vi "运维调试_采配水.vi"() -> ()   [LabVIEW 2016, in "PLC.lvlib"]
uses:
  PLC.lvlib
  <vilib>/Plasmionique/MB Master/MB_Master/MB_Master.lvclass
  <vilib>/Utility/miscctls.llb/LVPointTypeDef.ctl
  <vilib>/Plasmionique/MB Master/MB_Master_Serial/MB_Master_Serial.lvclass
  C:/Program Files (x86)/National Instruments/LabVIEW 2016/vi.lib/Plasmionique/MB Master/MB_Master/MB_Master.lvclass
  <vilib>/Plasmionique/MB Master/MB Master.lvlib
panel:
  out "R113":i16 caption="储水时间设定"
  out "R25":i16
  in  "V14NC":bool
  out "R24":i16
  in  "V14NO":bool
  out "X2":bool caption="X1"
  out "采配水版本号":string
  out "R23":i16 caption="清洗频次计数"
  out "R112":i16 caption="清洗频次设定"
  out "R22":i16
  in  "V13NC":bool
  out "R111":i16 caption="排液时间"
  out "通讯故障":bool
  out "R21":i16
  in  "V13NO":bool
  out "R20":i16
  in  "M1-2":bool
  in  "潜水泵工作模式":u16(ring) items=["泵1单泵单管路", "泵2单泵单管路", "双泵双管路"]
  out "X11":bool caption="废液报警"
  out "X10":bool caption="自来水检测"
  out "X9":bool caption="泵2过载报警"
  out "X8":bool caption="泵1过载报警"
  out "X7":bool caption="断电检测"
  out "X6":bool caption="开门检测"
  out "X5":bool caption="烟雾检测"
  out "X4":bool caption="漏水检测"
  out "X3":bool caption="进样检测"
  out "X1":bool
  out "X0":bool caption="采样池液位开关"
  out "R109":i16 caption="配水时间"
  out "集成报警信息":string
  out "R108":i16 caption="自来水报警"
  out "R107":i16 caption="采水池液位报警设置"
  out "R106":i16 caption="进样超时设置"
  out "R105":i16 caption="二级清洗时间"
  out "R104":i16 caption="一级清洗时间"
  out "R103":i16 caption="外部管路清洗时间"
  out "R102":i16 caption="静置沉淀时间"
  out "R101":i16 caption="内部管路润洗时间"
  out "R100":i16 caption="外部管路润洗时间"
  out "R2":i16
  out "R1":i16
  out "多列列表框":i32(listbox)
  out "R19":i16
  in  "V6":bool
  out "R18":i16
  in  "V5":bool
  out "R17":i16
  in  "V4":bool
  out "R16":i16
  in  "V3":bool
  out "R15":i16
  in  "V2":bool
  out "R14":i16
  in  "M2":bool
  out "R13":i16
  in  "V1":bool
  out "R12":i16
  in  "M1-1":bool
  in  "返回":bool
  in  "参数设置":bool
  in  "单步启动":bool
  in  "启动":bool
  in  "停止":bool
  # "S"
  # "次"
  # "次"
  # "S"
  # "S"
  # "S"
  # "S"
  # "S"
  # "S"
  # "S"
  # "S"
  # "S"
  # "S"
  # "S"
  # "单步计时："
  # "s"
  # "流程计时："
  # "s"
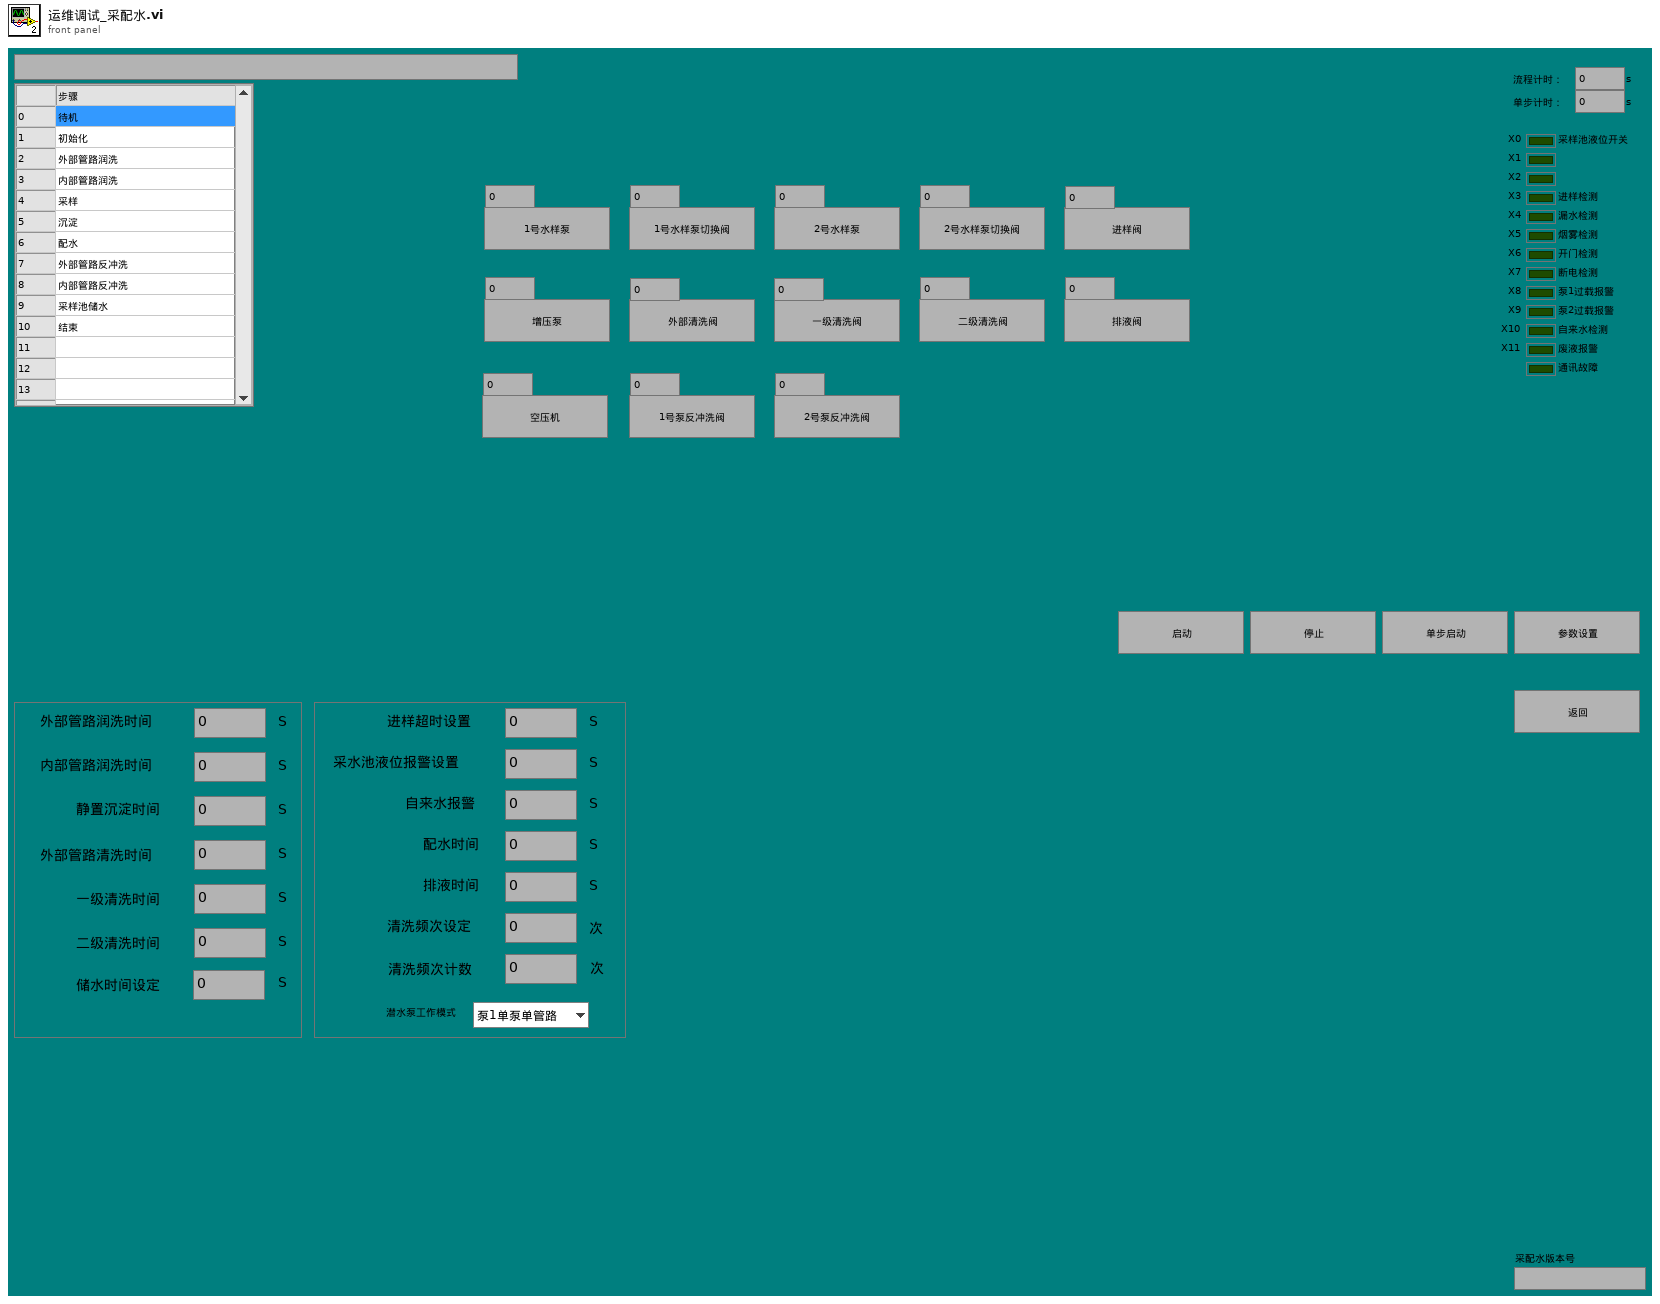
[diagram p1: front panel]
types:
  T1 = typedef "LVPointTypeDef.ctl" = cluster{"Horizontal":i16, "Vertical":i16}
  T2 = cluster{"时间标识":timestamp, "设备":string, "日志信息":string}
  T3 = cluster{"R0":i16, "R1":i16, "R2":i16, "R3":i16, "R4":i16, "R5":i16, "R6":i16, "R7":i16, "R8":i16, "R9":i16, "R10":i16, "R11":i16, "R12":i16, "R13":i16, "R14":i16, "R15":i16, "R16":i16, "R17":i16, "R18":i16, "R19":i16, "R20":i16, "R21":i16, "R22":i16, "R23":i16, "R24":i16, "R25":i16}
  T4 = cluster{"seconds since 1Jan1904":timestamp, "table输入":string, string, "table输入":string}
  T5 = cluster{"时间标识":timestamp, "设备":string, "日志信息":string, "流程参数":string}
  T6 = cluster{"命令":string, cluster{"starting address":u16, "holding register value":u16}}
  T7 = cluster{"CODCr":cluster{"启动测量模式":cluster{"测量模式":enum16{"水样测量", "标样核查", "零点核查", "加标回收", "平行样", "校零", "校标"}}, "确定按钮":bool}, "参数启用":cluster{"多参数":bool, "CODMn":bool, "总磷总氮":bool, "氨氮":bool, "CODcr":bool}}
  T8 = enum16{"水样测量", "标样核查", "零点核查", "加标回收", "平行样", "校零", "校标"}
  T9 = cluster{"命令":string, "数据":cluster{"starting address":u16, "holding register value":u16}}
  T10 = cluster{"命令":string, "数据":cluster{"starting address":u16, "holding register values":u16[]}}
  T11 = cluster{"命令":string, "data":cluster{"starting address":u16, "coil values":bool[]}}
  T12 = cluster{"多参数":bool, "CODMn":bool, "总磷总氮":bool, "氨氮":bool, "CODcr":bool}
  T13 = enum32{"Bad", "Idle", "Run top level", "Running"}
  T14 = cluster{"baud rate (bps)":u32, "stop bits":u16, "parity":u16, "flow control":u16, "timeout":u32, "retries":i32}
  T15 = cluster{"starting address":u16, "holding register values":u16[]}
  T16 = cluster{"starting address":u16, "holding register value":u16}
  T17 = cluster{"starting address":u16, "coil values":bool[]}
  T18 = cluster{"Registers[0]":u16, "Registers[1]":u16, "Registers[2]":u16, "Registers[3]":u16, "Registers[4]":u16, "Registers[5]":u16, "Registers[6]":u16, "Registers[7]":u16, "Registers[8]":u16, "Registers[9]":u16, "Registers[10]":u16, "Registers[11]":u16, "Registers[12]":u16, "Registers[13]":u16, "Registers[14]":u16, "Registers[15]":u16, "Registers[16]":u16, "Registers[17]":u16, "Registers[18]":u16, "Registers[19]":u16, "Registers[20]":u16, "Registers[21]":u16, "Registers[22]":u16, "Registers[23]":u16, "Registers[24]":u16, "Registers[25]":u16}
  T19 = cluster{"Registers[0]":u16, "Registers[1]":u16, "Registers[2]":u16, "Registers[3]":u16, "Registers[4]":u16, "Registers[5]":u16}
  T20 = cluster{"Registers[0]":u16, "Registers[1]":u16, "Registers[2]":u16, "Registers[3]":u16, "Registers[4]":u16, "Registers[5]":u16, "Registers[6]":u16, "Registers[7]":u16, "Registers[8]":u16, "Registers[9]":u16, "Registers[10]":u16, "Registers[11]":u16, "Registers[12]":u16, "Registers[13]":u16, "Registers[14]":u16, "Registers[15]":u16, "Registers[16]":u16, "Registers[17]":u16, "Registers[18]":u16, "Registers[19]":u16}
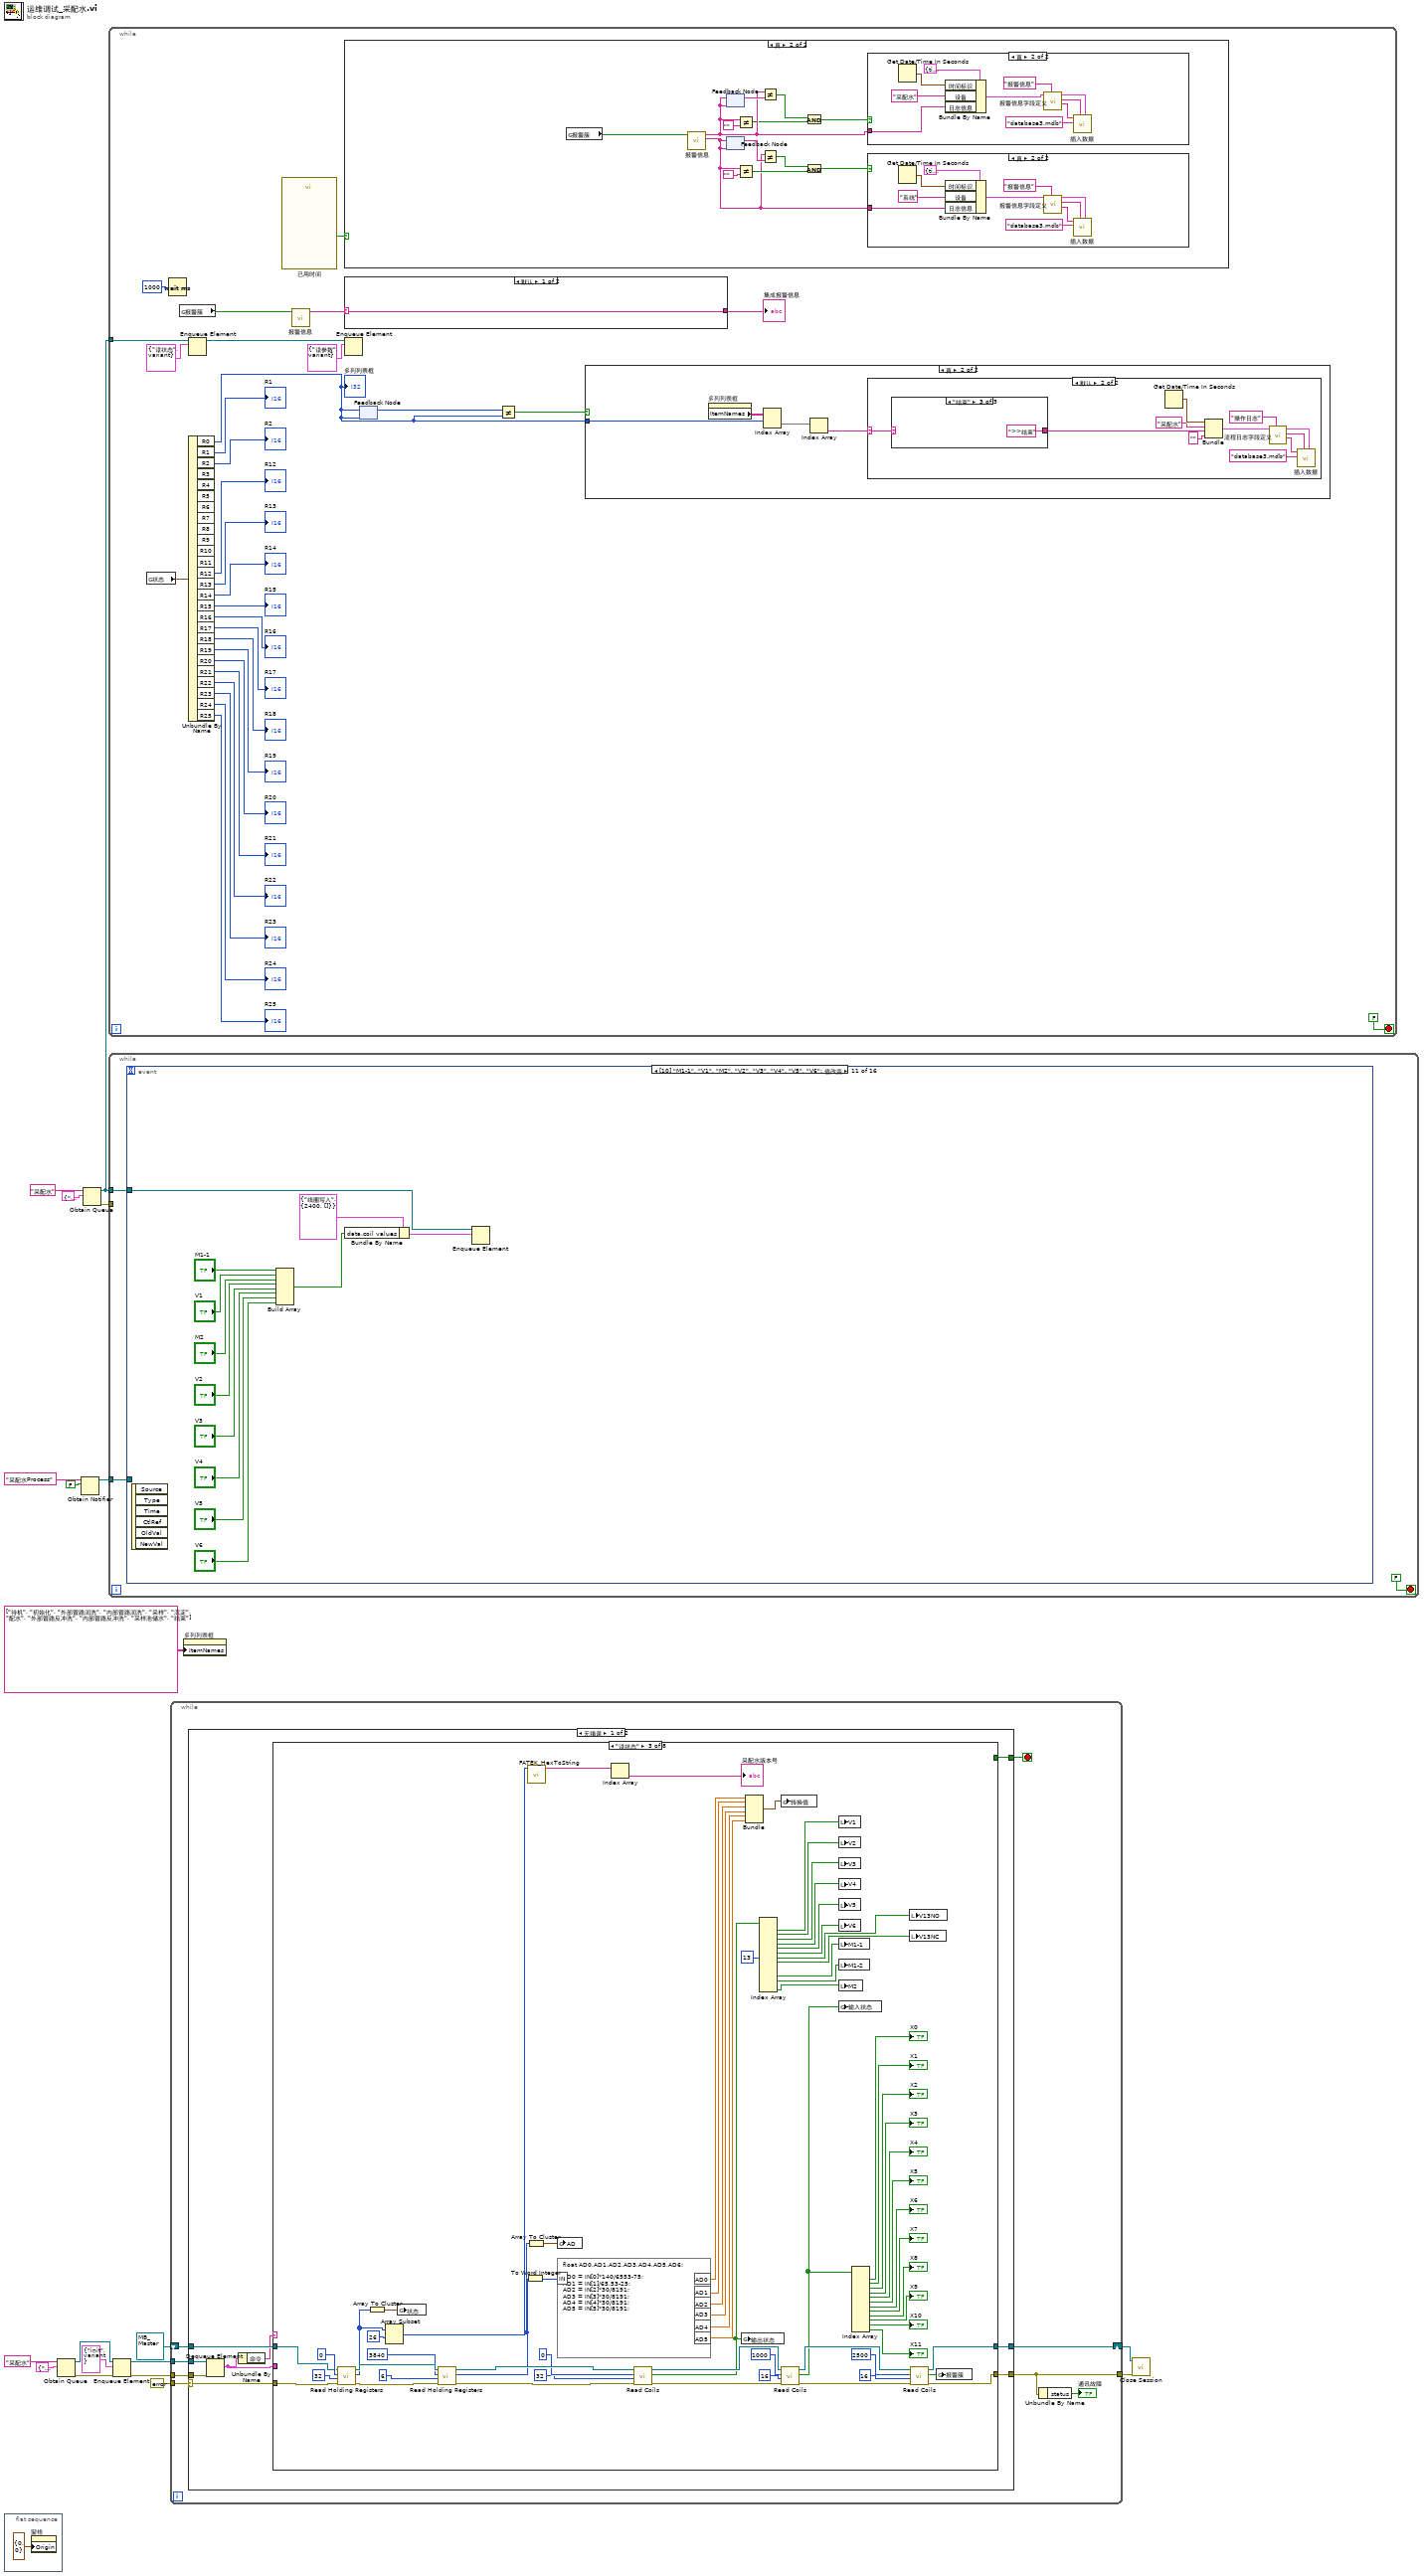
[diagram p0: block diagram]
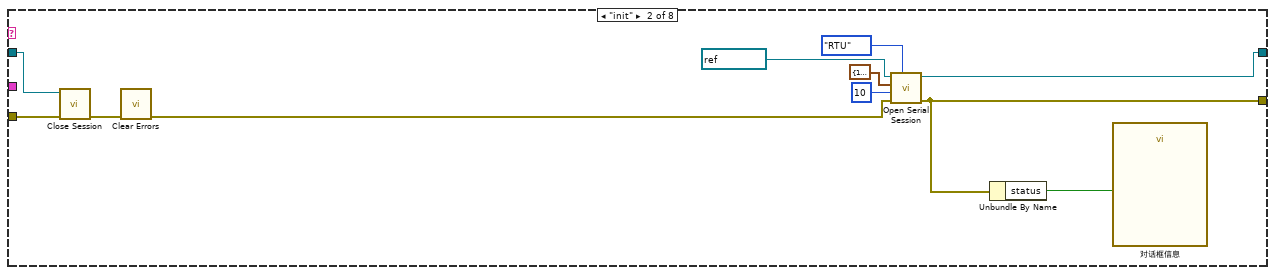
[diagram p3: hidden frame]
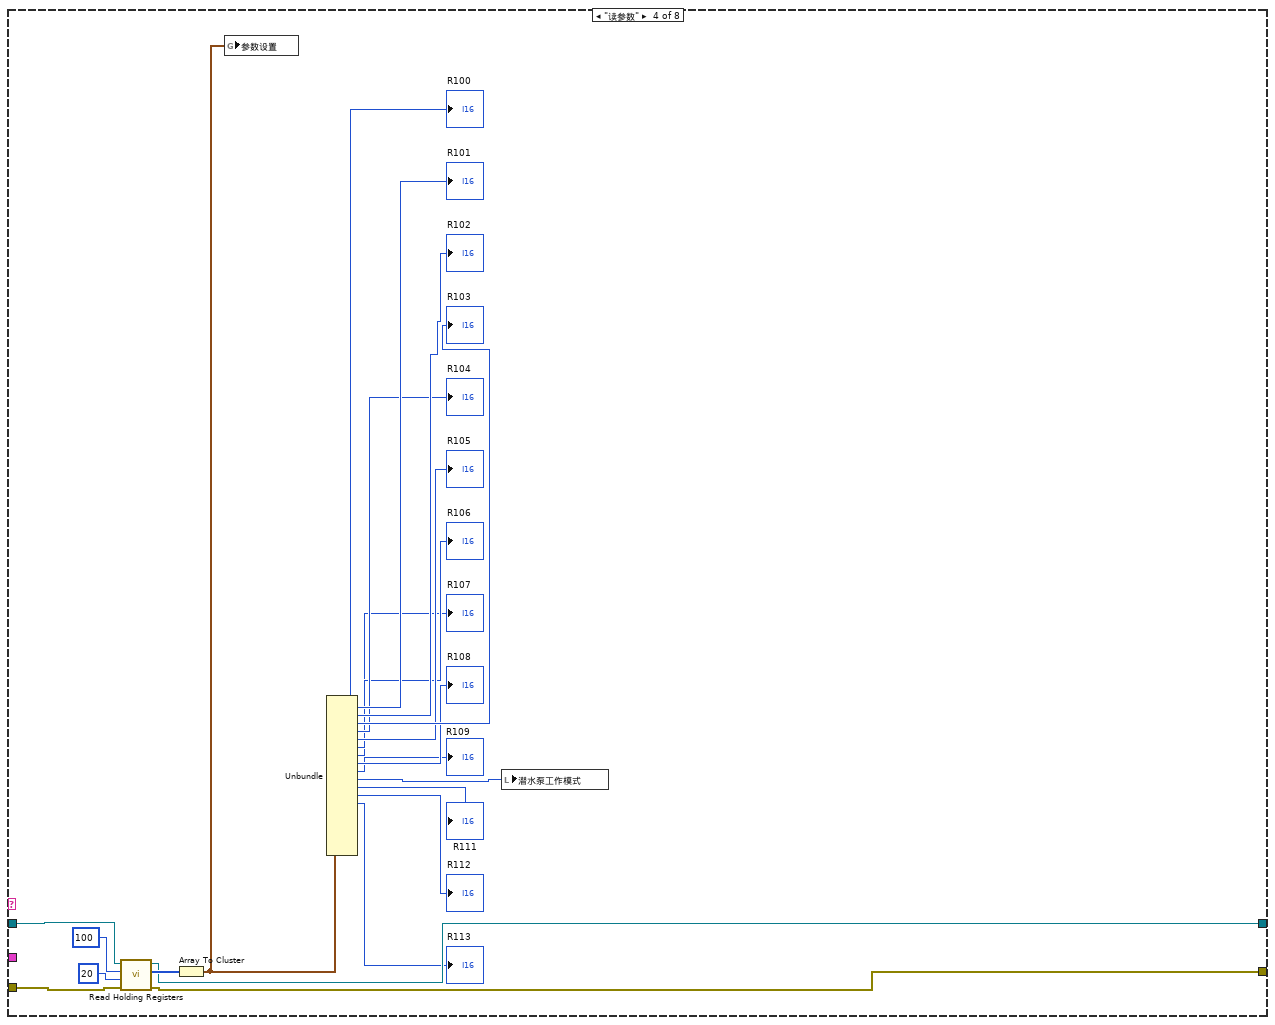
[diagram p4: hidden frame]
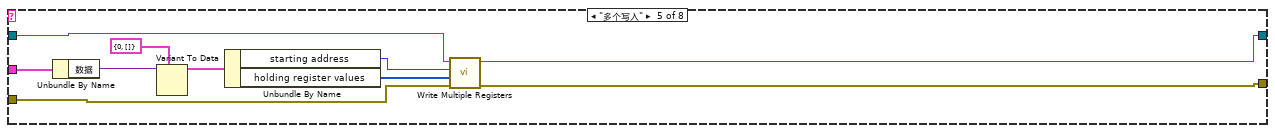
[diagram p5: hidden frame]
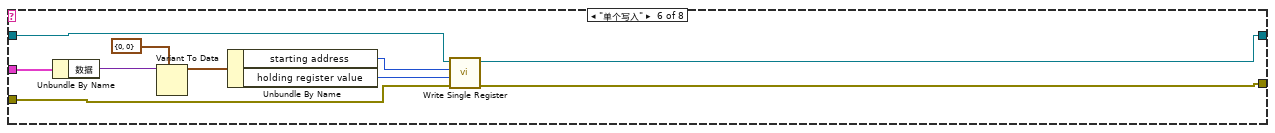
[diagram p6: hidden frame]
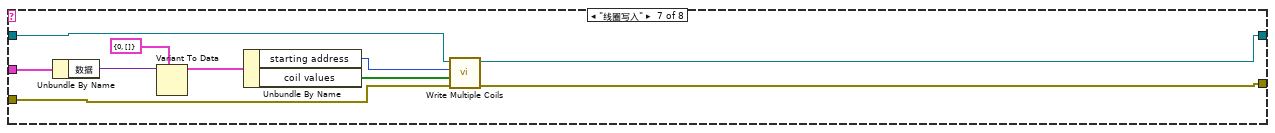
[diagram p7: hidden frame]
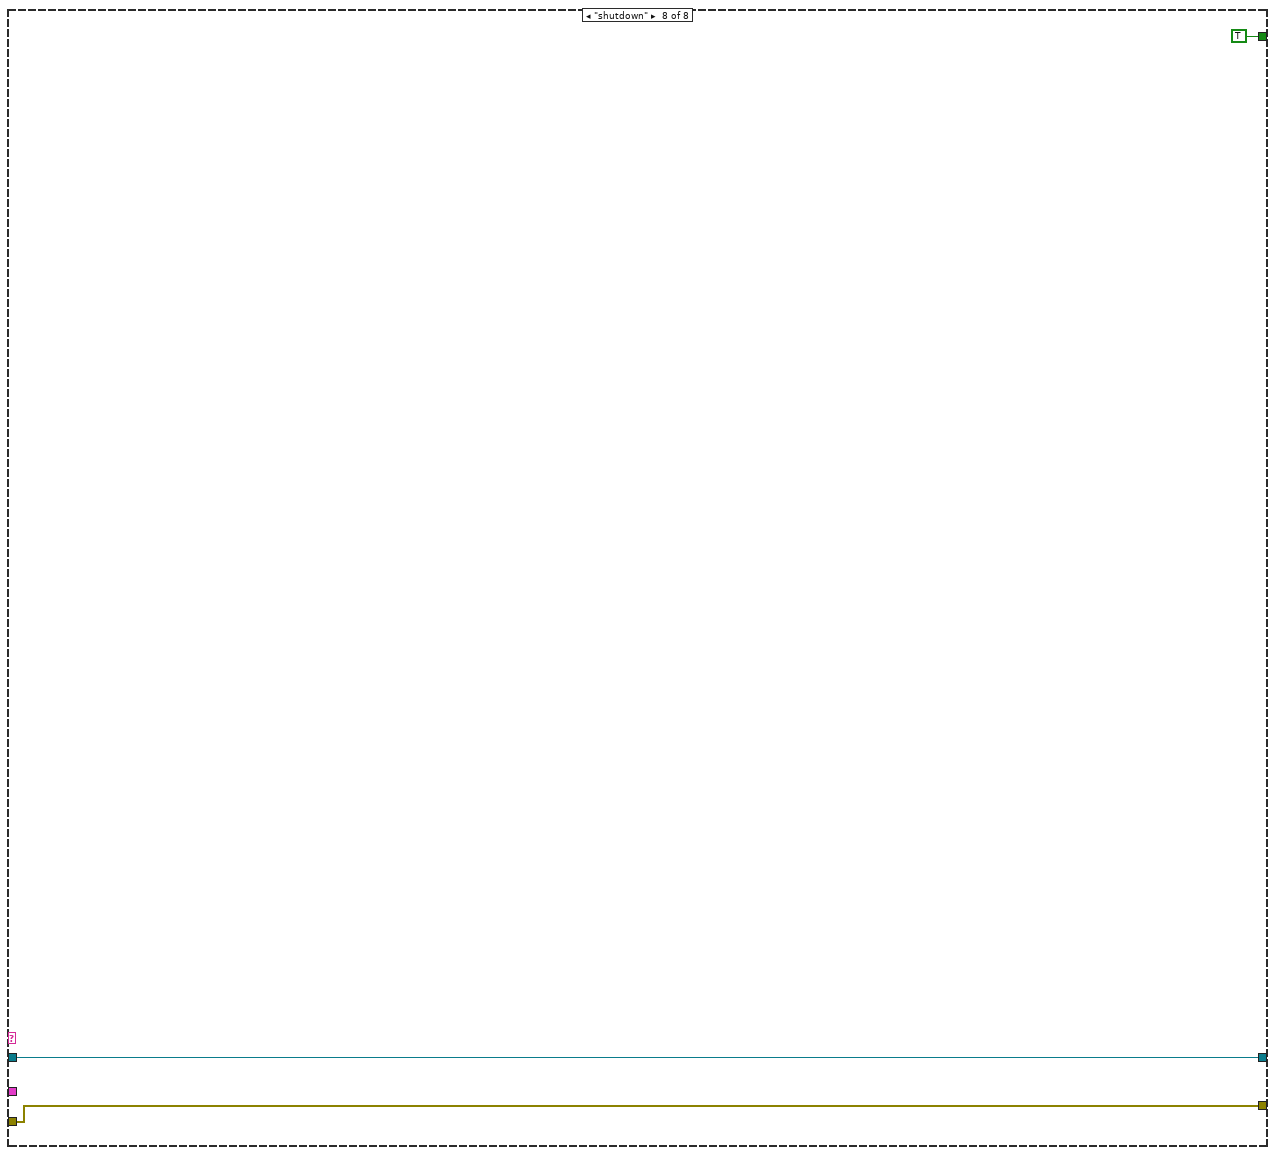
[diagram p8: hidden frame]
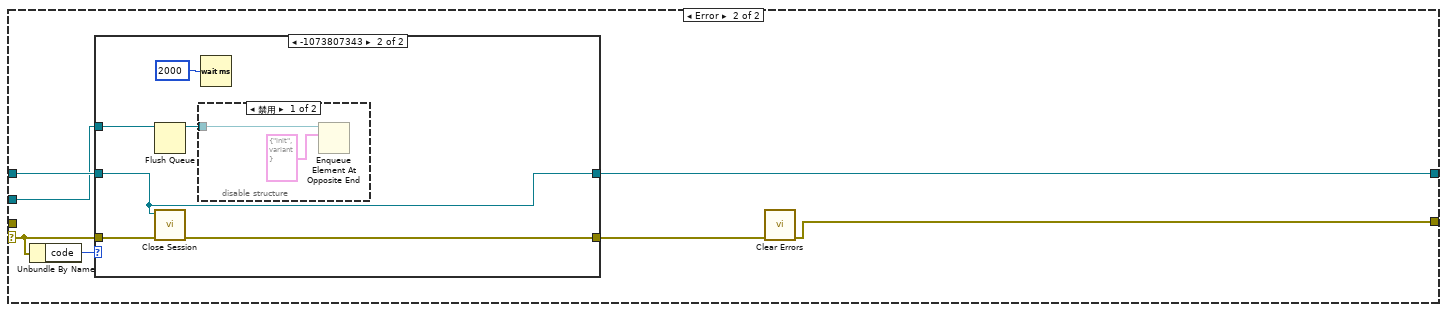
[diagram p9: hidden frame]
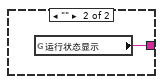
[diagram p15: hidden frame]
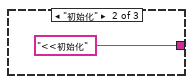
[diagram p19: hidden frame]
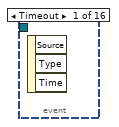
[diagram p20: hidden frame]
diagram:
  n1 = flat-sequence {
    frame #0 {
      n2 = property on="窗格" class="Pane"("Origin"=T1 {"Horizontal"=0, "Vertical"=0} ("原点")) -> ()  [unwired: 2 in, 2 out]
    }
  }
  n3 = Obtain Queue(name (unnamed)="采配水" ("名称（未命名）"), element data type=cluster{"命令":string, "数据":variant} {"命令"="", "数据"=variant}) -> (queue out=w9:refnum<queue>, error out=w8:errorcluster)  [unwired: 3 in, 1 out]
  n4 = Obtain Notifier(name (unnamed)="采配水Process" ("名称（未命名）"), notification data type=FALSE) -> (notifier out=w12:refnum<notifier>)  [unwired: 2 in, 2 out]
  n5 = Obtain Queue(name (unnamed)="采配水" ("名称（未命名）"), element data type=cluster{"命令":string, "数据":variant} {"命令"="", "数据"=variant}) -> (queue out=w16:refnum<queue>, error out=w17:errorcluster)  [unwired: 3 in, 1 out]
  n6 = while {
    tunnel: w16 -> [w49]
    stop <- FALSE stop-if-true
    n7 = global read "采配水全局变量.vi" "状态"() -> (w47:T3)
    n8 = Wait (ms)(milliseconds to wait=u32 1000 ("等待时间（毫秒）")) -> ()  [unwired: 1 out]
    n9 = global read "采配水全局变量.vi" "报警簇"() -> (w35:bool[])
    n10 = Enqueue Element(queue=w49, element=cluster{"命令":string, "数据":variant} {"命令"="读状态", "数据"=variant} ("元素")) -> (queue out=w30:refnum<queue>)  [unwired: 2 in, 2 out]
    n11 = Unbundle By Name(w47) -> ("R0"=w28:i16, "R1"=→"R1":i16, "R2"=→"R2":i16, "R12"=→"R12":i16, "R13"=→"R13":i16, "R14"=→"R14":i16, "R15"=→"R15":i16, "R16"=→"R16":i16, "R17"=→"R17":i16, "R18"=→"R18":i16, "R19"=→"R19":i16, "R20"=→"R20":i16, "R21"=→"R21":i16, "R22"=→"R22":i16, "R23"=→"R23":i16, "R24"=→"R24":i16, "R25"=→"R25":i16)  [unwired: 9 out]
    "多列列表框" <- w28
    n12 = call "已用时间"() -> ("Time has Elapsed"=w33:bool)  [unwired: 12 in, 7 out]
    n13 = call "报警信息.vi"("报警簇"=w35) -> ("采配水报警信息"=w27:string)  [unwired: 9 in, 1 out]
    n14 = case shown="真" w33 {
      frame False {
      }
      frame True {
        n15 = global read "采配水全局变量.vi" "报警簇"() -> (w63:bool[])
        n16 = call "报警信息.vi"("报警簇"=w63) -> ("系统报警信息"=w52:string, "采配水报警信息"=w59:string)  [unwired: 9 in]
        n17 = feedback #1(w59) -> (w62:string)
        n18 = feedback-in #1(w59) -> ()
        n19 = feedback #2(w52) -> (w53:string)
        n20 = feedback-in #2(w52) -> ()
        n21 = Not Equal?(x=w59, y="") -> (x != y?=w57:bool)
        n22 = Not Equal?(x=w52, y="") -> (x != y?=w56:bool)
        n23 = Not Equal?(x=w59, y=w62) -> (x != y?=w61:bool)
        n24 = Not Equal?(x=w52, y=w53) -> (x != y?=w54:bool)
        n25 = And(x=w61, y=w57) -> (x .and. y?=w60:bool)
        n26 = And(x=w54, y=w56) -> (x .and. y?=w51:bool)
        n27 = case shown="真" w60 {
          tunnel: w59 -> [_ w74]
          frame False {
          }
          frame True {
            n28 = Get Date/Time In Seconds() -> (seconds since 1Jan1904=w76:timestamp)
            n29 = Bundle By Name(cluster=T2 {"时间标识"=timestamp(0 s since 1904-01-01), "设备"="", "日志信息"=""} ("data in"), "时间标识"=w76, "设备"="采配水", "日志信息"=w74) -> (w77:T2)
            n30 = call "报警信息字段定义.vi"("table输入"="报警信息", "data in"=w77) -> ("table输出"=w81:string, "columns"=w82:string[], "data out"=w83:T2)  [unwired: 7 in]
            n31 = call "插入数据.vi"("data"=w83, "columns"=w82, "database"="database3.mdb", "table"=w81) -> ()  [unwired: 7 in, 1 out]
          }
        }
        n32 = case shown="真" w51 {
          tunnel: w52 -> [_ w64]
          frame False {
          }
          frame True {
            n33 = Get Date/Time In Seconds() -> (seconds since 1Jan1904=w66:timestamp)
            n34 = Bundle By Name(cluster=T2 {"时间标识"=timestamp(0 s since 1904-01-01), "设备"="", "日志信息"=""} ("data in"), "时间标识"=w66, "设备"="系统", "日志信息"=w64) -> (w67:T2)
            n35 = call "报警信息字段定义.vi"("table输入"="报警信息", "data in"=w67) -> ("table输出"=w71:string, "columns"=w72:string[], "data out"=w73:T2)  [unwired: 7 in]
            n36 = call "插入数据.vi"("data"=w73, "columns"=w72, "database"="database3.mdb", "table"=w71) -> ()  [unwired: 7 in, 1 out]
          }
        }
      }
    }
    n37 = case shown="默认" w27 {
      selector: w27 -> [w84 _]
      tunnel: [w84 w85] -> w34
      frame Default {
      }
      frame "" {
        n38 = global read "采配水全局变量.vi" "运行状态显示"() -> (w85:string)
      }
    }
    "集成报警信息" <- w34
    n39 = Enqueue Element(queue=w30, element=cluster{"命令":string, "数据":variant} {"命令"="读参数", "数据"=variant} ("元素")) -> ()  [unwired: 2 in, 3 out]
    n40 = feedback-in #3(w28) -> ()
    n41 = feedback #3(w28) -> (w29:i16)
    n42 = Not Equal?(x=w29, y=w28) -> (x != y?=w36:bool)
    n43 = case shown="真" w36 {
      tunnel: w28 -> [_ w88]
      frame False {
      }
      frame True {
        n44 = property on="多列列表框" class="MCListbox (严格)"() -> ("ItemNames"=w89:string[][])  [unwired: 2 in, 2 out]
        n45 = Index Array(array=w89, index (row)=w88) -> (element=w87:string[])  [unwired: 1 in]
        n46 = Index Array(array=w87) -> (element=w86:string)  [unwired: 1 in]
        n47 = case shown="默认" w86 {
          selector: w86 -> [_ w91]
          frame "待机" {
          }
          frame Default {
            n48 = case shown="\"结束\"" w91 {
              selector: w91 -> [w101 _ _]
              tunnel: [w101 "<<初始化" ">>结束"] -> w90
              frame Default {
              }
              frame "初始化" {
              }
              frame "结束" {
              }
            }
            n49 = Get Date/Time In Seconds() -> (seconds since 1Jan1904=w95:timestamp)
            n50 = Bundle("seconds since 1Jan1904"=w95, "table输入"="采配水", w90, "table输入"="") -> (w93:T4)  [unwired: 1 in]
            n51 = call "流程日志字段定义.vi"("table输入"="操作日志", "data in"=w93) -> ("table输出"=w98:string, "columns"=w99:string[], "data out"=w100:T5)  [unwired: 7 in]
            n52 = call "插入数据.vi"("data"=w100, "columns"=w99, "database"="database3.mdb", "table"=w98) -> ()  [unwired: 7 in, 1 out]
          }
        }
      }
    }
  }
  n53 = while {
    tunnel: w16 -> [w105]
    tunnel: w17 -> [_]
    tunnel: w12 -> [w104]
    stop <- FALSE stop-if-true
    n54 = event shown="[10] \"M1-1\", \"V1\", \"M2\", \"V2\", \"V3\", \"V4\", \"V5\", \"V6\": 值改变" {
      selector: _ -> [_ _ _ _ _ _ _ _ _ _ _ _ _ _ _ _]
      dyn-events: _ -> [_ _ _ _ _ _ _ _ _ _ _ _ _ _ _ _]
      timeout: _ -> [_ _ _ _ _ _ _ _ _ _ _ _ _ _ _ _]
      tunnel: w105 -> [_ w109 w112 w137 w156 w159 _ _ _ _ w187 w189 w194 w199 w204 w209]
      tunnel: w104 -> [_ w108 w111 _ _ _ _ _ _ _ _ _ _ _ _ _]
      event Timeout {
        n55 = event-data() -> ()  [unwired: 1 in, 3 out]
      }
      event "停止": Value Change {
        n56 = event-data() -> ()  [unwired: 1 in, 6 out]
        n57 = Send Notification(notification=TRUE ("通知"), notifier=w108) -> ()  [unwired: 1 in, 2 out]
        n58 = Enqueue Element At Opposite End(queue=w109, element=T6 {"命令"="单个写入", {"starting address"=300, "holding register value"=2}} ("元素")) -> ()  [unwired: 2 in, 3 out]
      }
      event "启动": Value Change {
        n59 = event-data() -> ()  [unwired: 1 in, 6 out]
        n60 = disable-structure shown="禁用" {
          disable-tunnel: w112 -> [w133 _]
          frame Disabled {
            n61 = Enqueue Element At Opposite End(queue=w133, element=T6 {"命令"="单个写入", {"starting address"=300, "holding register value"=1}} ("元素")) -> ()  [unwired: 2 in, 3 out]
          }
          frame Enabled {
          }
        }
        n62 = flat-sequence {
          tunnel: w111 -> [w113]
          frame #0 {
            n63 = Cancel Notification(0:w113) -> ()  [unwired: 1 in, 3 out]
          }
          frame #1 {
            n64 = call "手动启动选择对话框.vi"() -> ("确定"=w115:bool, "参数启用"=w114:T12)  [unwired: 10 in]
            n65 = case shown="真" w115 {
              tunnel: w114 -> [_ w116]
              frame False {
              }
              frame True {
                n66 = vi-ref "PLC.lvlib:一体站流程自动启动.vi"() -> (w119:refnum<vi>)
                n67 = property class="VI"(reference=w119) -> ("Name"=w118:string, "Exec.State"=w117:T13)  [unwired: 1 in, 2 out]
                n68 = case shown="\"Idle\"" w117 {
                  tunnel: w118 -> [_ w130 _ _]
                  tunnel: w116 -> [_ w120 _ _]
                  frame "Bad", Default {
                  }
                  frame "Idle" {
                    n69 = Bundle By Name(cluster=T7 {"CODCr"={"启动测量模式"={"测量模式"=enum."水样测量"}, "确定按钮"=FALSE}, "参数启用"={"多参数"=FALSE, "CODMn"=FALSE, "总磷总氮"=FALSE, "氨氮"=FALSE, "CODcr"=FALSE}} ("参数"), "CODCr.启动测量模式.测量模式"=T8."水样测量" ("CODMn.启动测量模式.测量模式"), "参数启用"=w120) -> (w121:T7)
                    n70 = Open VI Reference(type specifier VI Refnum (for type only)=refnum<vi> refnum, vi path=w130, options=128 ("选项")) -> (vi reference=w128:refnum<vi>, error out=w125:errorcluster)  [unwired: 3 in]
                    n71 = call-by-ref "开始异步调用"(reference=w128, error in=w125, "参数"=w121) -> (reference out=w126:refnum<vi>, error out=w124:errorcluster)  [unwired: 11 in]
                    n72 = Close Reference(reference=w126, error in (no error)=w124) -> ()  [unwired: 1 out]
                  }
                  frame "Run top level" {
                  }
                  frame "Running" {
                    n73 = One Button Dialog(message="流程已经运行,无须重复启动" ("消息")) -> ()  [unwired: 1 in, 1 out]
                  }
                }
              }
            }
          }
        }
      }
      event "单步启动": Value Change {
        n74 = event-data() -> ()  [unwired: 1 in, 6 out]
        n75 = call "单步启动对话框.vi"() -> ("单步启动步骤输出"=w134:u16)  [unwired: 11 in]
        n76 = Bundle By Name(cluster=T9 {"命令"="单个写入", "数据"={"starting address"=301, "holding register value"=0}} ("元素"), "数据.holding register value"=w134) -> (w135:T9)
        n77 = Enqueue Element At Opposite End(queue=w137, element=w135) -> ()  [unwired: 2 in, 3 out]
      }
      event "R100", "R101", "R102", "R103", "R104", "R105", "R106", "R107", "R108", "R109", "潜水泵工作模式", "R111", "R112", "R113": Value Change {
        n78 = event-data() -> ()  [unwired: 1 in, 6 out]
        n79 = local read "R100"() -> (w151:i16)
        n80 = local read "R101"() -> (w150:i16)
        n81 = local read "R102"() -> (w149:i16)
        n82 = local read "R103"() -> (w148:i16)
        n83 = local read "R104"() -> (w147:i16)
        n84 = local read "R105"() -> (w146:i16)
        n85 = local read "R106"() -> (w145:i16)
        n86 = local read "R107"() -> (w144:i16)
        n87 = local read "R108"() -> (w143:i16)
        n88 = local read "R109"() -> (w142:i16)
        n89 = local read "R111"() -> (w140:i16)
        n90 = local read "R112"() -> (w139:i16)
        n91 = local read "R113"() -> (w138:i16)
        n92 = Build Array(w151, w150, w149, w148, w147, w146, w145, w144, w143, w142, "潜水泵工作模式", w140, w139, w138) -> (w152:u16[])
        n93 = Bundle By Name(cluster=T10 {"命令"="多个写入", "数据"={"starting address"=0, "holding register values"=[]}} ("元素"), "数据.starting address"=u16 100, "数据.holding register values"=w152) -> (w153:T10)
        n94 = Enqueue Element At Opposite End(queue=w156, element=w153) -> ()  [unwired: 2 in, 3 out]
      }
      event "R23": Value Change {
        n95 = event-data() -> ()  [unwired: 1 in, 6 out]
        n96 = local read "R23"() -> (w158:i16)
        n97 = Build Array(w158) -> (w157:i16[])
        n98 = Bundle By Name(cluster=T10 {"命令"="多个写入", "数据"={"starting address"=0, "holding register values"=[]}} ("元素"), "数据.starting address"=u16 23, "数据.holding register values"=w157) -> (w160:T10)
        n99 = Enqueue Element At Opposite End(queue=w159, element=w160) -> ()  [unwired: 2 in, 3 out]
      }
      event "R23": Mouse Down {
        n100 = event-data() -> ("CtlRef"=w165:refnum<vi>)  [unwired: 1 in, 7 out]
        n101 = Two Button Dialog(message="请确认是否更改，更改后将影响实际清洗频次" ("消息")) -> (T button?=w164:bool)  [unwired: 2 in]
        n102 = case shown="真" w164 {
          tunnel: w165 -> [_ w166]
          frame False {
          }
          frame True {
            n103 = property class="DigNum (严格)"(reference=w166) -> (reference out=w168:refnum<vi>, "Value"=w169:i16)  [unwired: 1 in, 1 out]
            n104 = call "数字键盘.vi"("OldNumber"=w169) -> ("NewNumber"=w167:sgl)
            n105 = property class="DigNum (严格)"(reference=w168, "Val(Sgnl)"=w167) -> ()  [unwired: 1 in, 2 out]
          }
        }
      }
      event "R100", "R101", "R102", "R103", "R104", "R105", "R106", "R107", "R108", "R109", "R111", "R112", "R113": Mouse Down {
        n106 = event-data() -> ("CtlRef"=w173:refnum<vi>)  [unwired: 1 in, 7 out]
        n107 = property class="DigNum (严格)"(reference=w173) -> (reference out=w171:refnum<vi>, "Value"=w172:i16)  [unwired: 1 in, 1 out]
        n108 = call "数字键盘.vi"("OldNumber"=w172) -> ("NewNumber"=w170:sgl)
        n109 = property class="DigNum (严格)"(reference=w171, "Val(Sgnl)"=w170) -> ()  [unwired: 1 in, 2 out]
      }
      event "参数设置": Value Change {
        n110 = event-data() -> ()  [unwired: 1 in, 6 out]
        n111 = property on="窗格" class="Pane"("Origin"=T1 {"Horizontal"=0, "Vertical"=628} ("原点")) -> ()  [unwired: 2 in, 2 out]
      }
      event "返回": Value Change {
        n112 = event-data() -> ()  [unwired: 1 in, 6 out]
        n113 = property on="窗格" class="Pane"("Origin"=T1 {"Horizontal"=0, "Vertical"=0} ("原点")) -> ()  [unwired: 2 in, 2 out]
      }
      event "M1-1", "V1", "M2", "V2", "V3", "V4", "V5", "V6": Value Change {
        n114 = event-data() -> ()  [unwired: 1 in, 6 out]
        n115 = Build Array("M1-1", "V1", "M2", "V2", "V3", "V4", "V5", "V6") -> (w176:bool[])
        n116 = Bundle By Name(cluster=T11 {"命令"="线圈写入", "data"={"starting address"=2400, "coil values"=[]}} ("元素"), "data.coil values"=w176) -> (w177:T11)
        n117 = Enqueue Element(queue=w187, element=w177) -> ()  [unwired: 2 in, 3 out]
      }
      event "M1-2": Value Change {
        n118 = event-data() -> ()  [unwired: 1 in, 6 out]
        n119 = Build Array("M1-2") -> (w190:bool[])
        n120 = Bundle By Name(cluster=T11 {"命令"="线圈写入", "data"={"starting address"=2413, "coil values"=[]}} ("元素"), "data.coil values"=w190) -> (w191:T11)
        n121 = Enqueue Element(queue=w189, element=w191) -> ()  [unwired: 2 in, 3 out]
      }
      event "V13NO": Value Change {
        n122 = event-data() -> ()  [unwired: 1 in, 6 out]
        n123 = Build Array("V13NO") -> (w195:bool[])
        n124 = Bundle By Name(cluster=T11 {"命令"="线圈写入", "data"={"starting address"=2414, "coil values"=[]}} ("元素"), "data.coil values"=w195) -> (w196:T11)
        n125 = Enqueue Element(queue=w194, element=w196) -> ()  [unwired: 2 in, 3 out]
      }
      event "V13NC": Value Change {
        n126 = event-data() -> ()  [unwired: 1 in, 6 out]
        n127 = Build Array("V13NC") -> (w200:bool[])
        n128 = Bundle By Name(cluster=T11 {"命令"="线圈写入", "data"={"starting address"=2415, "coil values"=[]}} ("元素"), "data.coil values"=w200) -> (w201:T11)
        n129 = Enqueue Element(queue=w199, element=w201) -> ()  [unwired: 2 in, 3 out]
      }
      event "V14NO": Value Change {
        n130 = event-data() -> ()  [unwired: 1 in, 6 out]
        n131 = Build Array("V14NO") -> (w205:bool[])
        n132 = Bundle By Name(cluster=T11 {"命令"="线圈写入", "data"={"starting address"=2408, "coil values"=[]}} ("元素"), "data.coil values"=w205) -> (w206:T11)
        n133 = Enqueue Element(queue=w204, element=w206) -> ()  [unwired: 2 in, 3 out]
      }
      event "V14NC": Value Change {
        n134 = event-data() -> ()  [unwired: 1 in, 6 out]
        n135 = Build Array("V14NC") -> (w210:bool[])
        n136 = Bundle By Name(cluster=T11 {"命令"="线圈写入", "data"={"starting address"=2409, "coil values"=[]}} ("元素"), "data.coil values"=w210) -> (w211:T11)
        n137 = Enqueue Element(queue=w209, element=w211) -> ()  [unwired: 2 in, 3 out]
      }
    }
  }
  n138 = Enqueue Element(queue=w9, element=cluster{"命令":string, "数据":variant} {"命令"="init", "数据"=variant} ("元素"), error in (no error)=w8) -> (queue out=w4:refnum<queue>, error out=w6:errorcluster)  [unwired: 1 in, 1 out]
  n139 = while {
    tunnel: w4 -> [w217]
    tunnel: w6 -> [w216]
    shift-right: [w220] -> w1
    shift-left: refnum<class "MB_Master.lvclass"> refnum ("MB session in") -> [w219]
    tunnel: errorcluster {"status"=FALSE, "code"=0, "source"=""} ("error out") -> [w218]
    tunnel: [w214] -> w2
    stop <- w215 stop-if-true
    n140 = case shown="无错误" w218 {
      selector: w218 -> [w226 w367]
      tunnel: [w229 w366] -> w220
      tunnel: w219 -> [w228 w368]
      tunnel: [w227 w364] -> w214
      tunnel: w217 -> [w223 w363]
      tunnel: w216 -> [w222 _]
      tunnel: [w224 _] -> w215
      frame No Error {
        n141 = Dequeue Element(queue=w223, error in (no error)=w222) -> (element=w221:cluster{"命令":string, "数据":variant})  [unwired: 1 in, 3 out]
        n142 = Unbundle By Name(w221) -> ("命令"=w225:string)
        n143 = case shown="\"读状态\"" w225 {
          tunnel: [w231 w235 w277 w324 w336 w346 w356 w361] -> w229
          tunnel: w228 -> [w231 w239 w295 w329 w339 w349 w359 w361]
          tunnel: [w230 w237 w276 w323 w337 w347 w357 w360] -> w227
          tunnel: w226 -> [w230 w241 w298 w328 w338 w348 w358 w360]
          tunnel: [_ _ _ _ _ _ _ TRUE] -> w224
          tunnel: w221 -> [_ _ _ _ w335 w345 w355 _]
          frame "idle", Default {
          }
          frame "init" {
            n144 = call-dynamic "Close Session.vi"("error in (no error)"=w241, "MB session in"=w239) -> ("error out"=w240:errorcluster)  [unwired: 9 in]
            n145 = call <vilib>:"Clear Errors.vi"("error in (no error)"=w240) -> ("error out"=w238:errorcluster)  [unwired: 5 in, 1 out]
            n146 = call <vilib>:"Open Serial Session.vi"("Mode (RTU)"=enum16{"RTU", "ASCII"}."RTU", "Error in"=w238, "Slave ID"=u8 10, "Serial Config"=T14 {"baud rate (bps)"=115200, "stop bits"=10, "parity"=0, "flow control"=0, "timeout"=500, "retries"=1}, "VISA Resource"=refnum<visa-resource-name> "COM3" ("VISA resource name")) -> ("Error out"=w237:errorcluster, "MB_Serial session"=w235:refnum<class "MB_Master_Serial.lvclass">)  [unwired: 5 in]
            n147 = Unbundle By Name(w237) -> ("status"=w242:bool)
            n148 = call "对话框信息"("Enable"=w242) -> ()  [unwired: 9 in, 2 out]
          }
          frame "读状态" {
            n149 = call <vilib>:"Read Holding Registers.vi"("error in (no error)"=w298, "quantity"=u16 32 ("number of holding registers"), "starting address"=u16 0, "MB session in"=w295) -> ("error out"=w293:errorcluster, "Registers"=w262:u16[], "MB session out"=w294:refnum<class "MB_Master.lvclass">)  [unwired: 5 in]
            n150 = Array To Cluster(array=w262) -> (cluster=w299:T18)
            n151 = Array Subset(array=w262, index=26 ("索引")) -> (w260:u16[])  [unwired: 1 in]
            n152 = global write "采配水全局变量.vi" "状态"(w299) -> ()
            n153 = call <vilib>:"Read Holding Registers.vi"("error in (no error)"=w293, "quantity"=u16 6 ("number of holding registers"), "starting address"=u16 3840, "MB session in"=w294) -> ("error out"=w289:errorcluster, "Registers"=w264:u16[], "MB session out"=w290:refnum<class "MB_Master.lvclass">)  [unwired: 5 in]
            n154 = To Word Integer(number=w264) -> (16bit integer=w263:i16[])
            n155 = call "FATEK_HexToString.vi"("数组"=w260) -> ("STRING"=w259:string[])  [unwired: 10 in]
            n156 = Array To Cluster(array=w264) -> (cluster=w307:T19)
            n157 = global write "采配水全局变量.vi" "AD"(w307) -> ()
            n158 = formula code="float AD0,AD1,AD2,AD3,AD4,AD5,AD6;\n\nAD0 = IN[0]*140/6553-75;\nAD1 = IN[1]/65.53-25;\nAD2 = IN[2]*30/8191;\nAD3 = IN[3]*30/8191;\nAD4 = IN[4]*30/8191;\nAD5 = IN[5]*30/8191;"("IN"=w263) -> ("AD0"=w305:dbl, "AD1"=w304:dbl, "AD2"=w303:dbl, "AD3"=w302:dbl, "AD4"=w301:dbl, "AD5"=w300:dbl)
            n159 = Index Array(array=w259) -> (element=→"采配水版本号":string)  [unwired: 1 in]
            n160 = call <vilib>:"Read Coils.vi"("error in (no error)"=w289, "quantity"=u16 32 ("number of coils"), "starting address"=u16 0, "MB session in"=w290) -> ("error out"=w285:errorcluster, "Coils"=w268:bool[], "MB session out"=w286:refnum<class "MB_Master.lvclass">)  [unwired: 5 in]
            n161 = global write "采配水全局变量.vi" "输出状态"(w268) -> ()
            n162 = Bundle(w305, w304, w303, w302, w301, w300) -> (w306:cluster{dbl, dbl, dbl, dbl, dbl, dbl})  [unwired: 1 in]
            n163 = Index Array(array=w268, index #7=13 ("索引")) -> (element #1=w257:bool, element #2=w256:bool, element #3=w255:bool, element #4=w254:bool, element #5=w253:bool, element #6=w252:bool, element #7=w250:bool, element #8=w249:bool, element #11=w248:bool, element #12=w247:bool, element #14=w243:bool)  [unwired: 13 in, 3 out]
            n164 = global write "采配水全局变量.vi" "转换值"(w306) -> ()
            n165 = call <vilib>:"Read Coils.vi"("error in (no error)"=w285, "quantity"=u16 16 ("number of coils"), "starting address"=u16 1000, "MB session in"=w286) -> ("error out"=w281:errorcluster, "Coils"=w275:bool[], "MB session out"=w282:refnum<class "MB_Master.lvclass">)  [unwired: 5 in]
            n166 = local write "V1"(w257) -> ()
            n167 = local write "V2"(w256) -> ()
            n168 = local write "V3"(w255) -> ()
            n169 = local write "V4"(w254) -> ()
            n170 = local write "V5"(w253) -> ()
            n171 = local write "V6"(w252) -> ()
            n172 = local write "M1-1"(w248) -> ()
            n173 = local write "M1-2"(w247) -> ()
            n174 = local write "M2"(w243) -> ()
            n175 = global write "采配水全局变量.vi" "输入状态"(w275) -> ()
            n176 = Index Array(array=w275) -> (element #1=→"X0":bool, element #2=→"X1":bool, element #3=→"X2":bool, element #4=→"X3":bool, element #5=→"X4":bool, element #6=→"X5":bool, element #7=→"X6":bool, element #8=→"X7":bool, element #9=→"X8":bool, element #10=→"X9":bool, element #11=→"X10":bool, element #12=→"X11":bool)  [unwired: 12 in]
            n177 = local write "V13NO"(w250) -> ()
            n178 = local write "V13NC"(w249) -> ()
            n179 = call <vilib>:"Read Coils.vi"("error in (no error)"=w281, "quantity"=u16 16 ("number of coils"), "starting address"=u16 2500, "MB session in"=w282) -> ("error out"=w276:errorcluster, "Coils"=w278:bool[], "MB session out"=w277:refnum<class "MB_Master.lvclass">)  [unwired: 5 in]
            n180 = global write "采配水全局变量.vi" "报警簇"(w278) -> ()
          }
          frame "读参数" {
            n181 = call <vilib>:"Read Holding Registers.vi"("error in (no error)"=w328, "quantity"=u16 20 ("number of holding registers"), "starting address"=u16 100, "MB session in"=w329) -> ("error out"=w323:errorcluster, "Registers"=w325:u16[], "MB session out"=w324:refnum<class "MB_Master.lvclass">)  [unwired: 5 in]
            n182 = Array To Cluster(array=w325) -> (cluster=w312:T20)
            n183 = global write "采配水全局变量.vi" "参数设置"(w312) -> ()
            n184 = Unbundle(w312) -> ("Registers[0]"=→"R100":u16, "Registers[1]"=→"R101":u16, "Registers[2]"=→"R102":u16, "Registers[3]"=→"R103":u16, "Registers[4]"=→"R104":u16, "Registers[5]"=→"R105":u16, "Registers[6]"=→"R106":u16, "Registers[7]"=→"R107":u16, "Registers[8]"=→"R108":u16, "Registers[9]"=→"R109":u16, "Registers[10]"=w311:u16, "Registers[11]"=→"R111":u16, "Registers[12]"=→"R112":u16, "Registers[13]"=→"R113":u16)  [unwired: 6 out]
            n185 = local write "潜水泵工作模式"(w311) -> ()
          }
          frame "多个写入" {
            n186 = Unbundle By Name(w335) -> ("数据"=w334:variant)
            n187 = Variant To Data(type=T15 {"starting address"=0, "holding register values"=[]}, Variant=w334) -> (data=w332:T15)  [unwired: 1 in, 1 out]
            n188 = Unbundle By Name(w332) -> ("starting address"=w331:u16, "holding register values"=w330:u16[])
            n189 = call <vilib>:"Write Multiple Registers.vi"("error in (no error)"=w338, "values"=w330, "starting address"=w331, "MB session in"=w339) -> ("error out"=w337:errorcluster, "MB session out"=w336:refnum<class "MB_Master.lvclass">)  [unwired: 6 in]
          }
          frame "单个写入" {
            n190 = Unbundle By Name(w345) -> ("数据"=w344:variant)
            n191 = Variant To Data(type=T16 {"starting address"=0, "holding register value"=0}, Variant=w344) -> (data=w342:T16)  [unwired: 1 in, 1 out]
            n192 = Unbundle By Name(w342) -> ("starting address"=w341:u16, "holding register value"=w340:u16)
            n193 = call <vilib>:"Write Single Register.vi"("error in (no error)"=w348, "value"=w340, "address"=w341, "MB session in"=w349) -> ("error out"=w347:errorcluster, "MB session out"=w346:refnum<class "MB_Master.lvclass">)  [unwired: 6 in]
          }
          frame "线圈写入" {
            n194 = Unbundle By Name(w355) -> ("数据"=w354:variant)
            n195 = Variant To Data(type=T17 {"starting address"=0, "coil values"=[]}, Variant=w354) -> (data=w352:T17)  [unwired: 1 in, 1 out]
            n196 = Unbundle By Name(w352) -> ("starting address"=w351:u16, "coil values"=w350:bool[])
            n197 = call <vilib>:"Write Multiple Coils.vi"("error in (no error)"=w358, "values"=w350, "starting address"=w351, "MB session in"=w359) -> ("error out"=w357:errorcluster, "MB session out"=w356:refnum<class "MB_Master.lvclass">)  [unwired: 6 in]
          }
          frame "shutdown" {
          }
        }
      }
      frame Error {
        n198 = Unbundle By Name(w367) -> ("code"=w369:i32)
        n199 = case shown="-1073807343" w369 {
          tunnel: w368 -> [w371 w375]
          tunnel: w367 -> [w370 w377]
          tunnel: [w370 w376] -> w365
          tunnel: [w371 w375] -> w366
          tunnel: w363 -> [_ w374]
          frame Default {
          }
          frame -1073807343 {
            n200 = Flush Queue(queue=w374) -> (queue out=w373:refnum<queue>)  [unwired: 1 in, 2 out]
            n201 = call-dynamic "Close Session.vi"("error in (no error)"=w377, "MB session in"=w375) -> ("error out"=w376:errorcluster)  [unwired: 9 in]
            n202 = disable-structure shown="禁用" {
              disable-tunnel: w373 -> [w378 _]
              frame Disabled {
                n203 = Enqueue Element At Opposite End(queue=w378, element=cluster{"命令":string, "数据":variant} {"命令"="init", "数据"=variant} ("元素")) -> ()  [unwired: 2 in, 3 out]
              }
              frame Enabled {
              }
            }
            n204 = Wait (ms)(milliseconds to wait=u32 2000 ("等待时间（毫秒）")) -> ()  [unwired: 1 out]
          }
        }
        n205 = call <vilib>:"Clear Errors.vi"("error in (no error)"=w365) -> ("error out"=w364:errorcluster)  [unwired: 5 in, 1 out]
      }
    }
    n206 = Unbundle By Name(w214) -> ("status"=→"通讯故障":bool)
  }
  n207 = property on="多列列表框" class="MCListbox (严格)"("ItemNames"=string[][] [["待机"], ["初始化"], ["外部管路润洗"], ["内部管路润洗"], ["采样"], ["沉淀"], ["配水"], ["外部管路反冲洗"], ["内部管路反冲洗"], ["采样池储水"], ["结束"]] ("项名")) -> ()  [unwired: 2 in, 2 out]
  n208 = call-dynamic "Close Session.vi"("error in (no error)"=w2, "MB session in"=w1) -> ()  [unwired: 9 in, 1 out]
